vi "Simple TCP Server.vi"() -> ()   [LabVIEW 2023, in "VectoScratch.lvlib"]
uses:
  VectoScratch.lvlib
  Vecto/Connection State.ctl
  Vecto/proto/ConstellationCommand/Data.ctl
  Constellation Command Handler/Constellation Command Handler.lvclass/Constellation Command Handler.ctl
  Constellation Command Handler/Constellation Command Handler.lvclass
  C:/Users/zcoll/Documents/constellation/lv-vecto/Vecto/TCPMessageHandler/TCPMessageHandler.lvclass
  C:/Users/zcoll/Documents/constellation/lv-vecto/Vecto/TCPConnectionHandler/TCPConnectionHandler.lvclass
  Vecto/SequenceCountService/SequenceCountService.lvclass
  Vecto/TCPMessaging/TCPMessaging.lvclass
  Vecto/Vecto.lvlib
  Vecto/proto/ConstellationCommand/ConstellationCommand.lvlib
panel:
  in  "Server Stop":bool
  out "Command":T1 {"Time Stamp" format="%<%x %.3X>T"}
  out "error out":errorcluster
  out "Server State":T2=enum."Disconnected"
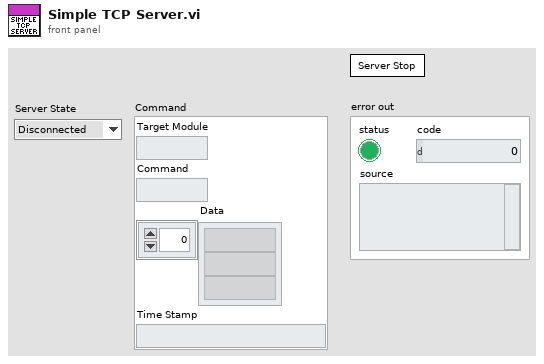
[diagram p1: front panel]
types:
  T1 = typedef "ConstellationCommand.lvlib/Data.ctl" = cluster{"Target Module":string, "Command":string, "Data":string[], "Time Stamp":timestamp}
  T2 = typedef "Vecto.lvlib/Connection State.ctl" = enum16{"Connected", "Disconnected"}
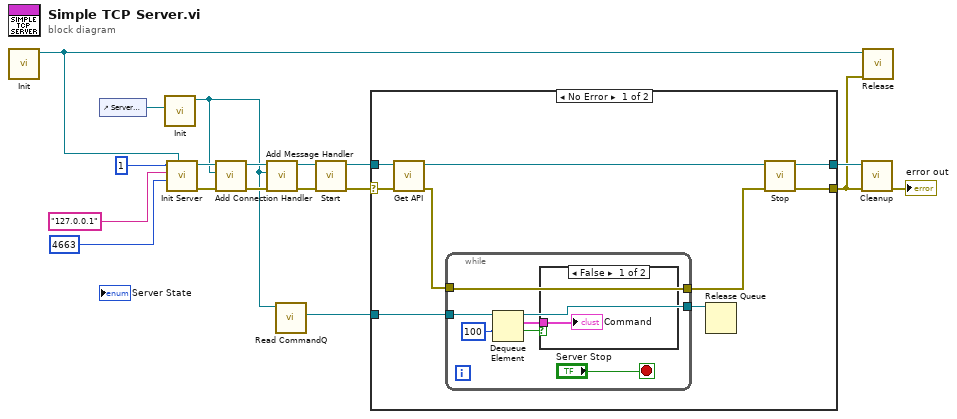
[diagram p0: block diagram]
diagram:
  n1 = call "Init.vi"() -> ("SequenceCountService out"=w7:refnum<class "SequenceCountService.lvclass">)  [unwired: 10 in, 1 out]
  n2 = control-ref of="Server State"() -> (w3:refnum<vi>)
  n3 = call "Init.vi"("State"=w3) -> ("Constellation Command Handler out"=w2:refnum<class "Constellation Command Handler.lvclass">)  [unwired: 10 in]
  n4 = call "Init Server.vi"("SequenceCountService"=w7, "Bind Port"=u16 4663 ("Remote Port"), "Bind Address"="127.0.0.1" ("Remote Address"), "Node ID"=u32 1) -> ("error out"=w8:errorcluster, "TCPMessaging out"=w9:refnum<class "TCPMessaging.lvclass">)  [unwired: 6 in]
  n5 = call "Add Connection Handler.vi"("error in (no error)"=w8, "TCPConnectionHandler"=w2, "TCPMessaging in"=w9) -> ("error out"=w12:errorcluster, "TCPMessaging out"=w17:refnum<class "TCPMessaging.lvclass">)  [unwired: 7 in]
  n6 = call "Add Message Handler.vi"("error in (no error)"=w12, "TCPMessageHandler"=w2, "TCPMessaging in"=w17) -> ("error out"=w11:errorcluster, "TCPMessaging out"=w18:refnum<class "TCPMessaging.lvclass">)  [unwired: 7 in]
  n7 = call "Read CommandQ.vi"("Constellation Command Handler in"=w2) -> ("CommandQ"=w1:refnum<queue>)  [unwired: 9 in, 1 out]
  n8 = call "Start.vi"("error in (no error)"=w11, "TCPMessaging in"=w18) -> ("error out"=w16:errorcluster, "TCPMessaging out"=w15:refnum<class "TCPMessaging.lvclass">)  [unwired: 8 in]
  n9 = case shown="No Error" w16 {
    selector: w16 -> [w26 w36]
    tunnel: w15 -> [w27 w37]
    tunnel: [w24 w37] -> w14
    tunnel: [w23 w36] -> w13
    tunnel: w1 -> [w22 _]
    frame No Error {
      n10 = call "Get API.vi"("error in (no error)"=w26, "TCPMessaging in"=w27) -> ("error out"=w21:errorcluster, "TCPMessaging out"=w25:refnum<class "TCPMessaging.lvclass">)  [unwired: 7 in, 1 out]
      n11 = while {
        tunnel: w22 -> [w34]
        tunnel: w21 -> [w32]
        tunnel: [w32] -> w20
        tunnel: [w30] -> w19
        stop <- "Server Stop" stop-if-true
        n12 = Dequeue Element(queue=w34, timeout in ms (-1)=100) -> (queue out=w30:refnum<queue>, element=w33:T1, timed out?=w28:bool)  [unwired: 1 in, 1 out]
        n13 = case shown="False" w28 {
          tunnel: w33 -> [w35 _]
          frame False {
            "Command" <- w35
          }
          frame True {
          }
        }
      }
      n14 = Release Queue(queue=w19) -> ()  [unwired: 2 in, 3 out]
      n15 = call "Stop.vi"("error in (no error)"=w20, "TCPMessaging in"=w25) -> ("error out"=w23:errorcluster, "TCPMessaging out"=w24:refnum<class "TCPMessaging.lvclass">)  [unwired: 8 in]
    }
    frame Error {
    }
  }
  n16 = call "Cleanup.vi"("error in (no error)"=w13, "TCPMessaging in"=w14) -> ("error out"=→"error out":errorcluster)  [unwired: 9 in]
  n17 = call "Release.vi"("error in (no error)"=w13, "SequenceCountService in"=w7) -> ()  [unwired: 9 in, 1 out]
